vi "Write Header - GUI Data.vi"(8 "error in (no error)":errorcluster, 11 "Save Image in":refnum<class "Save Image.lvclass">) -> (0 "error out":errorcluster, 3 "Save Image out":refnum<class "Save Image.lvclass">)   [LabVIEW 2018, in "Save Image.lvclass"]
uses:
  Save Image.lvclass
  TCS_ACS/TCS_ACS.lvclass
  <vilib>/Utility/Data Type/NI_Data Type.lvlib
  Simulated_Header/Simulated_Header.lvclass
  Simulated_Header/write keyword - integer.vi
  Simulated_Header/write keyword - boolean.vi
  Simulated_Header/write keyword - string.vi
  Simulated_Header/write keyword - float.vi
panel:
  out "Header parameters":T1
  out "TCS parameters":T2
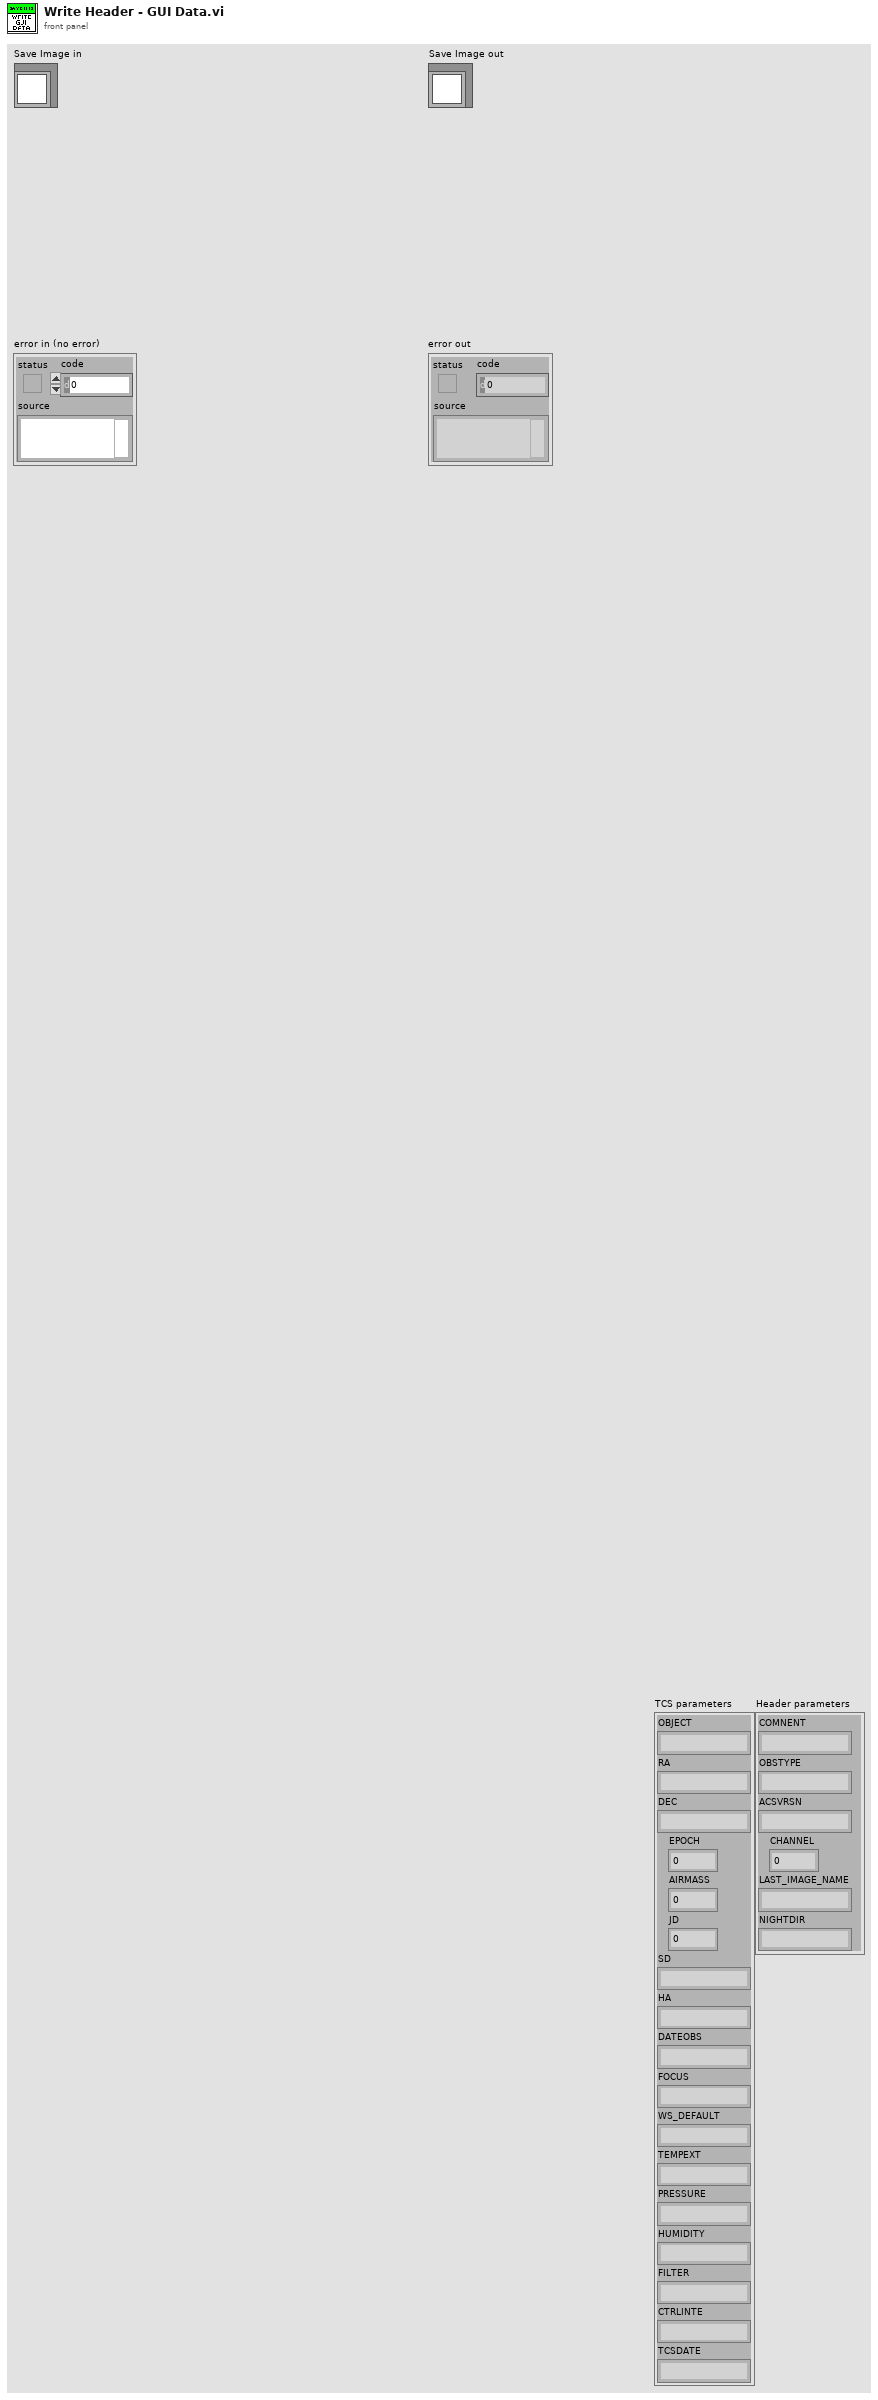
[diagram p1: front panel]
types:
  T1 = cluster{"COMNENT":string, "OBSTYPE":string, "ACSVRSN":string, "CHANNEL":u16, "LAST_IMAGE_NAME":string, "NIGHTDIR":string}
  T2 = cluster{"OBJECT":string, "RA":string, "DEC":string, "EPOCH":dbl, "AIRMASS":dbl, "JD":dbl, "SD":string, "HA":string, "DATEOBS":string, "FOCUS":string, "WS_DEFAULT":string, "TEMPEXT":string, "PRESSURE":string, "HUMIDITY":string, "FILTER":string, "CTRLINTE":string, "TCSDATE":string}
  T3 = cluster{"OBJ":string, "RA":string, "DEC":string, "EPOCH":dbl, "AIRMASS":dbl, "JD":dbl, "SD":string, "HA":string, "DATEOBS":string, "FOCUS":string, "WS_DEFAULT":string, "TEMP":string, "BAR":string, "HUM":string, "FILTER":string, "CTRLINTE":string, "TCSDATE":string}
  T4 = typedef "NI_Data Type.lvlib/Data Type.ctl" = enum8{"Invalid Type", "Void", "I8", "I16", "I32", "I64", "U8", "U16", "U32", "U64", "Single Float", "Double Float", "Extended Float", "Single Complex", "Double Complex", "Extended Complex", "Enum U8", "Enum U16", "Enum U32", "Enum U64", "Single Float With Unit", "Double Float With Unit", "Extended Float With Unit", "Single Complex with Unit", "Double Complex with Unit", "Extended Complex with Unit", "Boolean", "String", "Path", "Picture", "Tag", "Array", "Cluster", "Variant", "LV Variant", "Waveform", "Timestamp", "Digital Waveform", "Digital Data", "ExpressData", "Refnum", "External Data", "VI", "Poly VI", "LabVIEW Class Instance", "Fixed Point"}
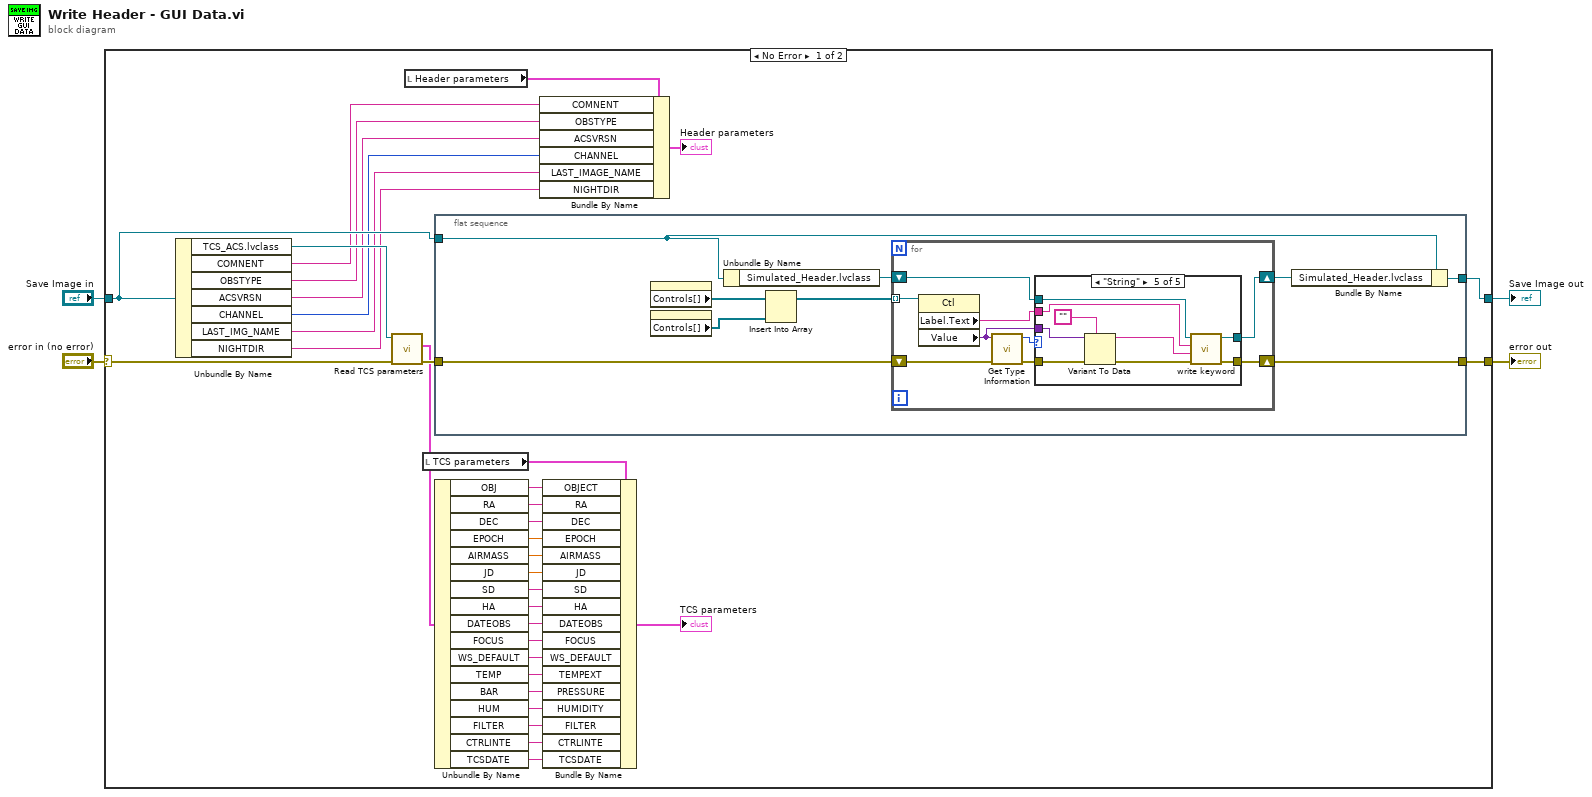
[diagram p0: block diagram]
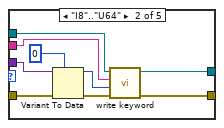
[diagram p3: hidden frame]
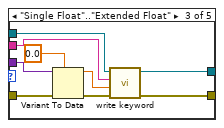
[diagram p4: hidden frame]
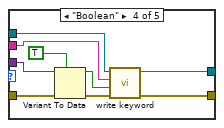
[diagram p5: hidden frame]
diagram:
  n1 = case shown="No Error" "error in (no error)" {
    selector: "error in (no error)" -> [w37 w95]
    tunnel: [w34 w95] -> w3
    tunnel: [w5 w96] -> w1
    tunnel: "Save Image in" -> [w36 w96]
    frame No Error {
      n2 = Unbundle By Name(w36) -> ("TCS_ACS.lvclass"=w38:refnum<class "TCS_ACS.lvclass">, "COMNENT"=w31:string, "OBSTYPE"=w30:string, "ACSVRSN"=w29:string, "CHANNEL"=w28:u16, "LAST_IMG_NAME"=w27:string, "NIGHTDIR"=w26:string)
      n3 = call "Read TCS parameters.vi"("error in (no error)"=w37, "TCS_ACS in"=w38) -> ("error out"=w35:errorcluster, "TCS parameters"=w23:T3)  [unwired: 7 in, 1 out]
      n4 = local read "Header parameters"() -> (w33:T1)
      n5 = local read "TCS parameters"() -> (w25:T2)
      n6 = flat-sequence {
        tunnel: [w47] -> w5
        tunnel: w36 -> [w40]
        tunnel: w35 -> [w45]
        tunnel: [w44] -> w34
        frame #0 {
          n7 = property on="TCS parameters" class="Clust (strict)"() -> ("Controls[]"=w43:refnum<vi>[])  [unwired: 2 in, 2 out]
          n8 = property on="Header parameters" class="Clust (strict)"() -> ("Controls[]"=w42:refnum<vi>[])  [unwired: 2 in, 2 out]
          n9 = Unbundle By Name(w40) -> ("Simulated_Header.lvclass"=w39:refnum<class "Simulated_Header.lvclass">)
          n10 = Insert Into Array(array=w43, new element=w42) -> (w41:refnum<vi>[])  [unwired: 1 in]
          n11 = for {
            shift-right: [w50] -> w46
            shift-left: w39 -> [w48]
            shift-right: [w51] -> w44
            shift-left: w45 -> [w55]
            tunnel: w41 -> [w56] mode=indexing
            n12 = property class="Ctl"(reference=w56) -> ("Label.Text"=w52:string, "Value"=w49:variant)  [unwired: 1 in, 2 out]
            n13 = call <vilib>:"Get Type Information.vi"("error in (no error)"=w55, "Variant"=w49) -> ("error out"=w53:errorcluster, "Type"=w54:T4)  [unwired: 5 in, 3 out]
            n14 = case shown="\"String\"" w54 {
              tunnel: w53 -> [w57 w67 w76 w85 w94]
              tunnel: w52 -> [_ w63 w72 w81 w90]
              tunnel: w48 -> [w58 w62 w71 w80 w89]
              tunnel: [w57 w61 w70 w79 w88] -> w51
              tunnel: [w58 w60 w69 w78 w87] -> w50
              tunnel: w49 -> [_ w59 w68 w77 w86]
              frame "Invalid Type", Default {
              }
              frame "I8".."U64" {
                n15 = Variant To Data(error in=w67, type=0, Variant=w59) -> (data=w64:i32, error out=w65:errorcluster)
                n16 = call-poly "write keyword.vi"("error in (no error)"=w65, "Value"=w64, "keyword"=w63, "Simulated_Header in"=w62) -> ("error out"=w61:errorcluster, "Simulated_Header out"=w60:refnum<class "Simulated_Header.lvclass">)  [unwired: 6 in]
              }
              frame "Single Float".."Extended Float" {
                n17 = Variant To Data(error in=w76, type=0.0, Variant=w68) -> (data=w73:dbl, error out=w74:errorcluster)
                n18 = call-poly "write keyword.vi"("error in (no error)"=w74, "Value"=w73, "keyword"=w72, "Simulated_Header in"=w71) -> ("error out"=w70:errorcluster, "Simulated_Header out"=w69:refnum<class "Simulated_Header.lvclass">)  [unwired: 6 in]
              }
              frame "Boolean" {
                n19 = Variant To Data(error in=w85, type=TRUE, Variant=w77) -> (data=w82:bool, error out=w83:errorcluster)
                n20 = call-poly "write keyword.vi"("error in (no error)"=w83, "value"=w82, "keyword"=w81, "Simulated_Header in"=w80) -> ("error out"=w79:errorcluster, "Simulated_Header out"=w78:refnum<class "Simulated_Header.lvclass">)  [unwired: 6 in]
              }
              frame "String" {
                n21 = Variant To Data(error in=w94, type="", Variant=w86) -> (data=w91:string, error out=w92:errorcluster)
                n22 = call-poly "write keyword.vi"("error in (no error)"=w92, "value"=w91, "keyword"=w90, "Simulated_Header in"=w89) -> ("error out"=w88:errorcluster, "Simulated_Header out"=w87:refnum<class "Simulated_Header.lvclass">)  [unwired: 6 in]
              }
            }
          }
          n23 = Bundle By Name(cluster=w40, "Simulated_Header.lvclass"=w46) -> (w47:refnum<class "Save Image.lvclass">)
        }
      }
      n24 = Unbundle By Name(w23) -> ("OBJ"=w6:string, "RA"=w7:string, "DEC"=w8:string, "EPOCH"=w9:dbl, "AIRMASS"=w10:dbl, "JD"=w11:dbl, "SD"=w12:string, "HA"=w13:string, "DATEOBS"=w14:string, "FOCUS"=w15:string, "WS_DEFAULT"=w16:string, "TEMP"=w17:string, "BAR"=w18:string, "HUM"=w19:string, "FILTER"=w20:string, "CTRLINTE"=w21:string, "TCSDATE"=w22:string)
      n25 = Bundle By Name(cluster=w33, "COMNENT"=w31, "OBSTYPE"=w30, "ACSVRSN"=w29, "CHANNEL"=w28, "LAST_IMAGE_NAME"=w27, "NIGHTDIR"=w26) -> (→"Header parameters":T1)
      n26 = Bundle By Name(cluster=w25, "OBJECT"=w6, "RA"=w7, "DEC"=w8, "EPOCH"=w9, "AIRMASS"=w10, "JD"=w11, "SD"=w12, "HA"=w13, "DATEOBS"=w14, "FOCUS"=w15, "WS_DEFAULT"=w16, "TEMPEXT"=w17, "PRESSURE"=w18, "HUMIDITY"=w19, "FILTER"=w20, "CTRLINTE"=w21, "TCSDATE"=w22) -> (→"TCS parameters":T2)
    }
    frame Error {
    }
  }
  "error out" <- w3
  "Save Image out" <- w1
